vi "AutoPlayParser.vi"(0 "Auto Play":string) -> (1 "Drive Command Strings":string[](array[string]), 2 "Drive Parameter Strings":string[](array[string]), 3 "Manipulator Command Strings":string[](array[string]), 4 "Manipulator Parameter Strings":string[](array[string]))   [LabVIEW 2020]
doc: "This VI parses a FRC 4265 standard autonomous play into two parallel sequences of steps and parameter strings. One sequence commands the robot's drive base while the other sequence commands the robot manipulator subsytems."
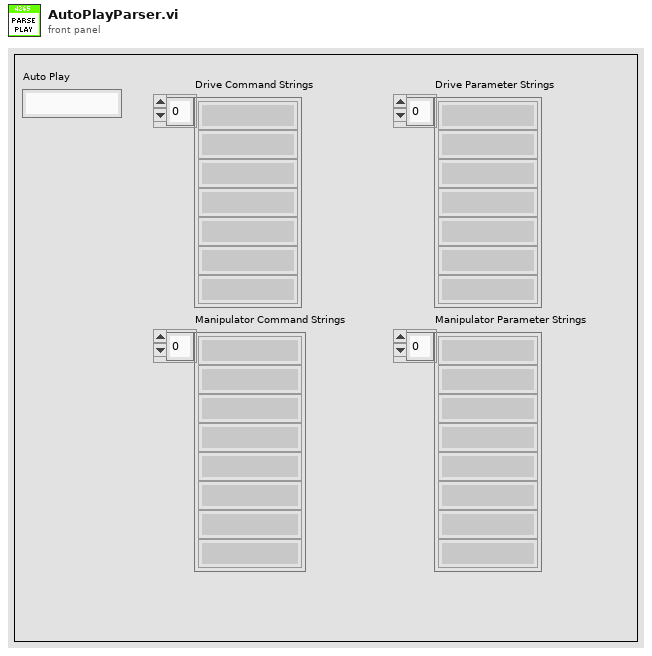
[diagram p1: front panel]
types:
  T1 = enum16{"Native", "Native Command Line", "UNIX", "Macintosh", "DOS"}
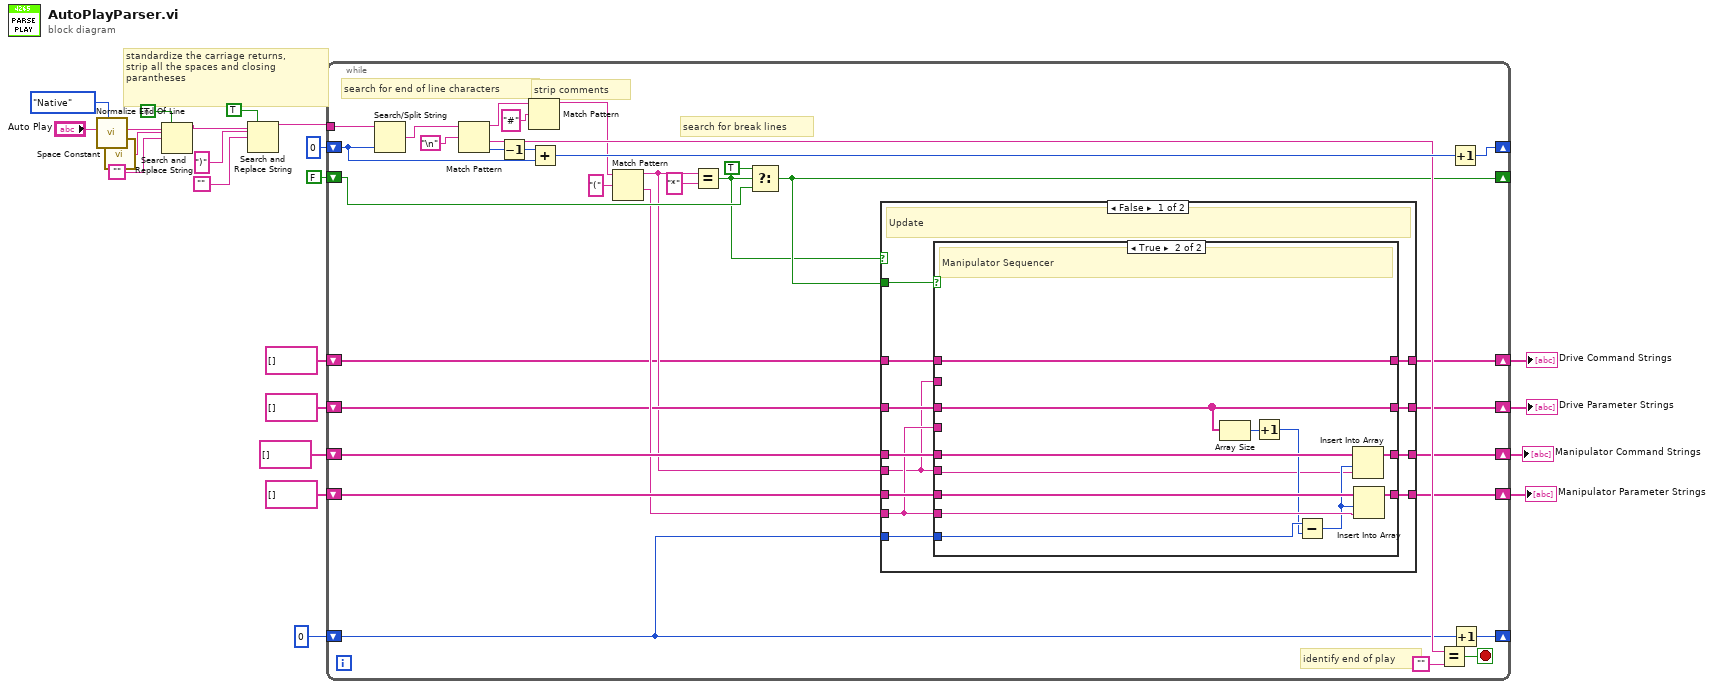
[diagram p0: block diagram]
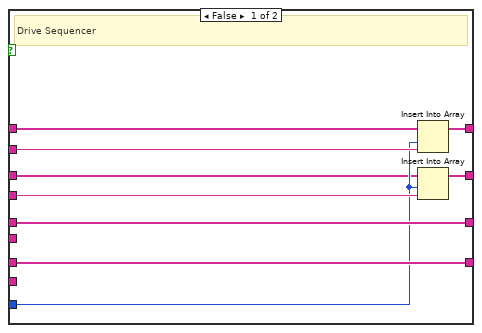
[diagram p2: hidden frame]
diagram:
  # "standardize the carriage returns, \nstrip all the spaces and closing\nparantheses"
  n1 = call <vilib>:"Normalize End Of Line.vi"("end of line (Native)"=T1."Native", "string in"="Auto Play") -> ("string out"=w9:string)  [unwired: 6 in]
  n2 = call <vilib>:"Space Constant.vi"() -> ("String"=w8:string)
  n3 = Search and Replace String(replace all?=TRUE ("replace all? (F)"), input string=w9, search string=w8, replace string="") -> (result string=w3:string)  [unwired: 4 in, 3 out]
  n4 = Search and Replace String(replace all?=TRUE ("replace all? (F)"), input string=w3, search string=")", replace string="") -> (result string=w2:string)  [unwired: 4 in, 3 out]
  n5 = while {
    tunnel: w2 -> [w52]
    shift-right: [w47] -> _
    shift-left: 0 ("offset (0)") -> [w49]
    shift-right: [w44] -> _
    shift-left: 0 -> [w36]
    shift-right: [w43] -> w12
    shift-left: string[] [] -> [w42]
    shift-right: [w41] -> w20
    shift-left: string[] [] -> [w40]
    shift-right: [w35] -> _
    shift-left: FALSE -> [w37]
    shift-right: [w33] -> w18
    shift-left: string[] [] -> [w32]
    shift-right: [w30] -> w17
    shift-left: string[] [] -> [w29]
    stop <- w53 stop-if-true
    # "identify end of play"
    # "search for break lines"
    # "search for end of line characters"
    # "strip comments"
    n6 = Search/Split String(string=w52, offset (0)=w49) -> (match + rest of string=w51:string)  [unwired: 1 in, 2 out]
    n7 = Match Pattern(string=w51, regular expression="\n") -> (before substring=w25:string, after substring=w46:string, offset past match=w50:i32)  [unwired: 1 in, 1 out]
    n8 = Decrement(x=w50) -> (x-1=w26:i32)
    n9 = Match Pattern(string=w25, regular expression="#") -> (before substring=w24:string)  [unwired: 1 in, 3 out]
    n10 = Add(x=w26, y=w49) -> (x+y=w48:i32)
    n11 = Match Pattern(string=w24, regular expression="(") -> (before substring=w31:string, after substring=w34:string)  [unwired: 1 in, 2 out]
    n12 = Equal?(x=w31, y="*") -> (x = y?=w28:bool)
    n13 = Select(t=TRUE, s=w28, f=w37) -> (s? t:f=w35:bool)
    n14 = case shown="False" w28 {
      tunnel: [w66 w89] -> w43
      tunnel: w42 -> [w65 w89]
      tunnel: [w64 w88] -> w41
      tunnel: w40 -> [w63 w88]
      tunnel: w36 -> [w62 _]
      tunnel: w35 -> [w61 _]
      tunnel: w34 -> [w60 _]
      tunnel: [w59 w90] -> w33
      tunnel: w32 -> [w58 w90]
      tunnel: w31 -> [w57 _]
      tunnel: [w56 w91] -> w30
      tunnel: w29 -> [w55 w91]
      frame False {
        # "Update"
        n15 = case shown="True" w61 {
          tunnel: [w75 w87] -> w66
          tunnel: w65 -> [w75 w86]
          tunnel: w60 -> [_ w85]
          tunnel: [w74 w84] -> w64
          tunnel: w63 -> [w74 w83]
          tunnel: w57 -> [_ w76]
          tunnel: w62 -> [w68 w80]
          tunnel: w60 -> [w73 _]
          tunnel: [w72 w81] -> w59
          tunnel: w58 -> [w67 w81]
          tunnel: w57 -> [w71 _]
          tunnel: [w70 w82] -> w56
          tunnel: w55 -> [w69 w82]
          frame False {
            # "Drive Sequencer"
            n16 = Insert Into Array(array=w69, index=w68, new element=w71) -> (w70:string[])
            n17 = Insert Into Array(array=w67, index=w68, new element=w73) -> (w72:string[])
          }
          frame True {
            # "Manipulator Sequencer"
            n18 = Array Size(array=w81) -> (size(s)=w79:i32)
            n19 = Increment(x=w79) -> (x+1=w77:i32)
            n20 = Subtract(x=w80, y=w77) -> (x-y=w78:i32)
            n21 = Insert Into Array(array=w86, index=w78, new element=w76) -> (w87:string[])
            n22 = Insert Into Array(array=w83, index=w78, new element=w85) -> (w84:string[])
          }
        }
      }
      frame True {
        # "Skip Break Line"
      }
    }
    n23 = Equal?(x=w46, y="") -> (x = y?=w53:bool)
    n24 = Increment(x=w48) -> (x+1=w47:i32)
    n25 = Increment(x=w36) -> (x+1=w44:i32)
  }
  "Manipulator Parameter Strings" <- w20
  "Drive Parameter Strings" <- w18
  "Drive Command Strings" <- w17
  "Manipulator Command Strings" <- w12
